vi "SpreadsheetRead.vi"() -> ()   [LabVIEW 2015]
uses:
  <vilib>/Utility/file.llb/Read Delimited Spreadsheet (DBL).vi
panel:
  out "Output Cluster":cluster{"X Array":dbl[], "Y Array":dbl[]}
  out "Acceleration Curve":cluster{"all rows":dbl[], "all rows":dbl[]}(graph)
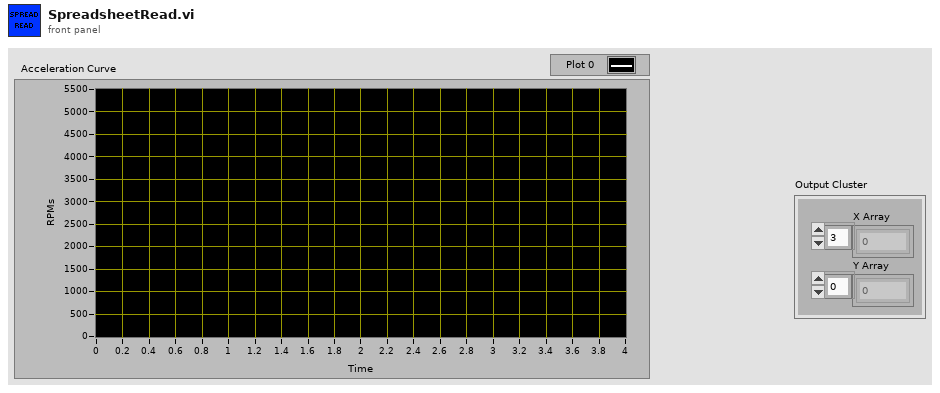
[diagram p1: front panel]
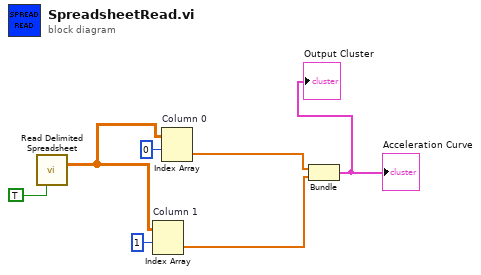
[diagram p0: block diagram]
diagram:
  n1 = call-poly <vilib>:"Read Delimited Spreadsheet.vi"("transpose? (F)"=TRUE) -> ("all rows"=w5:dbl[][])  [unwired: 9 in, 5 out]
  n2 = Index Array "Column 1"(array=w5, index (row)=1 ("index")) -> (element=w3:dbl[])  [unwired: 1 in]
  n3 = Index Array "Column 0"(array=w5, index (row)=0 ("index")) -> (element=w4:dbl[])  [unwired: 1 in]
  n4 = Bundle("all rows"=w4, "all rows"=w3) -> (→"Acceleration Curve" →"Output Cluster":cluster{"all rows":dbl[], "all rows":dbl[]})  [unwired: 1 in]
